vi "Write Experiment VariablesV2.vi"(8 "error in (no error)":errorcluster, 10 "Experiment Variables":T2={"DC_Bias"=0.0, "StartFreq"=0.0, "Duration"=0.0, "State"=enum."Initialization", "window ratio"=0.0, "Final Freq"=0.0}, 11 "ChirpV2 in":refnum<class "ChirpV2.lvclass">) -> (0 "error out":errorcluster, 3 "ChirpV2 out":refnum<class "ChirpV2.lvclass">)   [LabVIEW 2014, in "ChirpV2.lvclass"]
uses:
  ChirpV2.lvclass
  StateV2.ctl
  ChirpV2.lvclass/ChirpV2.ctl
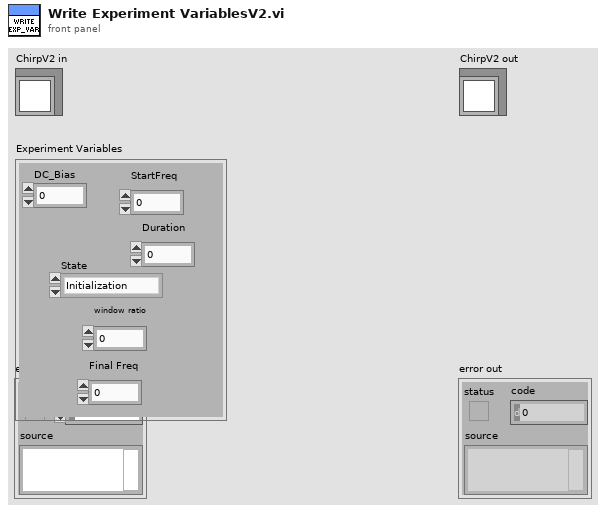
[diagram p1: front panel]
types:
  T1 = typedef "ChirpV2.lvclass/StateV2.ctl" = enum16{"WaitDC", "Initialization", "ChirpSetUp", "Wait", "ChirpMeasurement", "DFT", "WriteData", "Queue", "Ternimation"}
  T2 = cluster{"DC_Bias":dbl, "StartFreq":dbl, "Duration":dbl, "State":T1, "window ratio":dbl, "Final Freq":dbl}
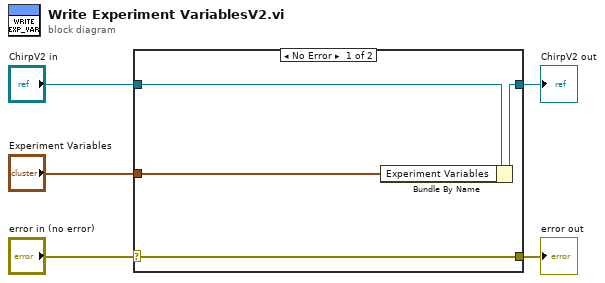
[diagram p0: block diagram]
diagram:
  n1 = case shown="No Error" "error in (no error)" {
    selector: "error in (no error)" -> [w9 w10]
    tunnel: [w9 w10] -> w4
    tunnel: [w7 w11] -> w2
    tunnel: "ChirpV2 in" -> [w8 w11]
    tunnel: "Experiment Variables" -> [w6 _]
    frame No Error {
      n2 = Bundle By Name(cluster=w8, "Experiment Variables"=w6) -> (w7:refnum<class "ChirpV2.lvclass">)
    }
    frame Error {
    }
  }
  "error out" <- w4
  "ChirpV2 out" <- w2
